vi "Set Station Time V.vi"(8 "error in (no error)":errorcluster, 11 "para0":T1) -> (0 "error out":errorcluster, 2 "function return":i16, 3 "para0 out":T1)   [LabVIEW 2009, in "VantagePro.lvlib"]
doc: "DllAccess short int _stdcall SetStationTime_V (DateTimeStamp *);"
uses:
  VantagePro.lvlib
  <userlib>/VantagePro/VantagePro.dll
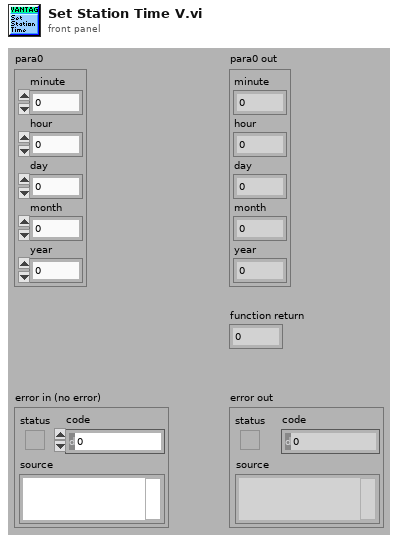
[diagram p1: front panel]
types:
  T1 = cluster{"minute":i32, "hour":i32, "day":i32, "month":i32, "year":i32}
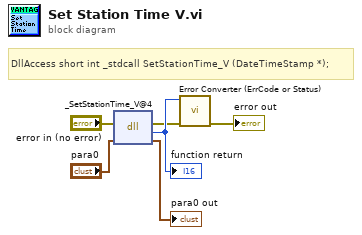
[diagram p0: block diagram]
diagram:
  # "DllAccess short int _stdcall SetStationTime_V (DateTimeStamp *);"
  n1 = dll-call lib="C:/Program Files/National Instruments/LabVIEW 2010/user.lib/VantagePro/VantagePro.*" fn="_SetStationTime_V@4"(error in="error in (no error)", "para0"="para0") -> (error out=w2:errorcluster, w6:i16, "para0"=→"para0 out":T1)  [unwired: 2 in, 1 out]
  "function return" <- w6
  n2 = call "Error Converter (ErrCode or Status).vi"("error in (no error)"=w2, "error code"=w6) -> ("error out"=→"error out":errorcluster)  [unwired: 9 in]
